vi "Display.vi"(8 "error in":errorcluster, 11 "Custom - Two Button in":refnum<class "Custom - Two Button.lvclass">) -> (0 "error out":errorcluster, 3 "Custom - Two Button out":refnum<class "Custom - Two Button.lvclass">)   [LabVIEW 2021, in "Pop-Up.lvlib" / "Custom - Two Button.lvclass"]
doc: "This VI will display a custom image to the user along with their message and buttons for pos/neg choice\n\n<b>Code Developed By:</b>\nDaniel Coons\nTechnology Service Corporation\n1983 S Liberty Drive\nBloomington, IN 47403\nPhone: 812 558-7100\ndaniel.coons@tsc.com\nwww.tsc.com/atcs"
uses:
  Custom - Two Button.lvclass
  C:/Development/Open Source/tsc-pop-up/Popup/Popup.lvclass
  <vilib>/Utility/miscctls.llb/LVPositionTypeDef.ctl
  Custom - Two Button.lvclass/Custom - Two Button.ctl
  Popup/Popup.lvclass/Popup.ctl
  Popup/Data Member Access/Read Theme.vi
  Theme/Theme.lvclass
  Popup/Popup.lvclass
  user32.dll
panel:
  out "header":bool
  in  "n-choice":bool
  in  "y-choice":bool
  out "2D Picture":picture
  out "Message":string
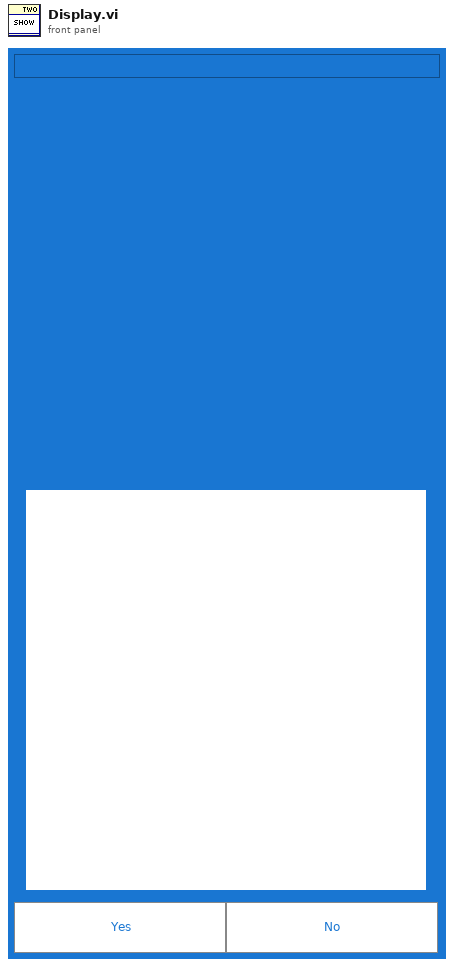
[diagram p1: front panel]
types:
  T1 = typedef "LVPositionTypeDef.ctl" = cluster{"Left":i32, "Top":i32}
  T2 = typedef "LVPoint32TypeDef.ctl" = cluster{"Horizontal":i32, "Vertical":i32}
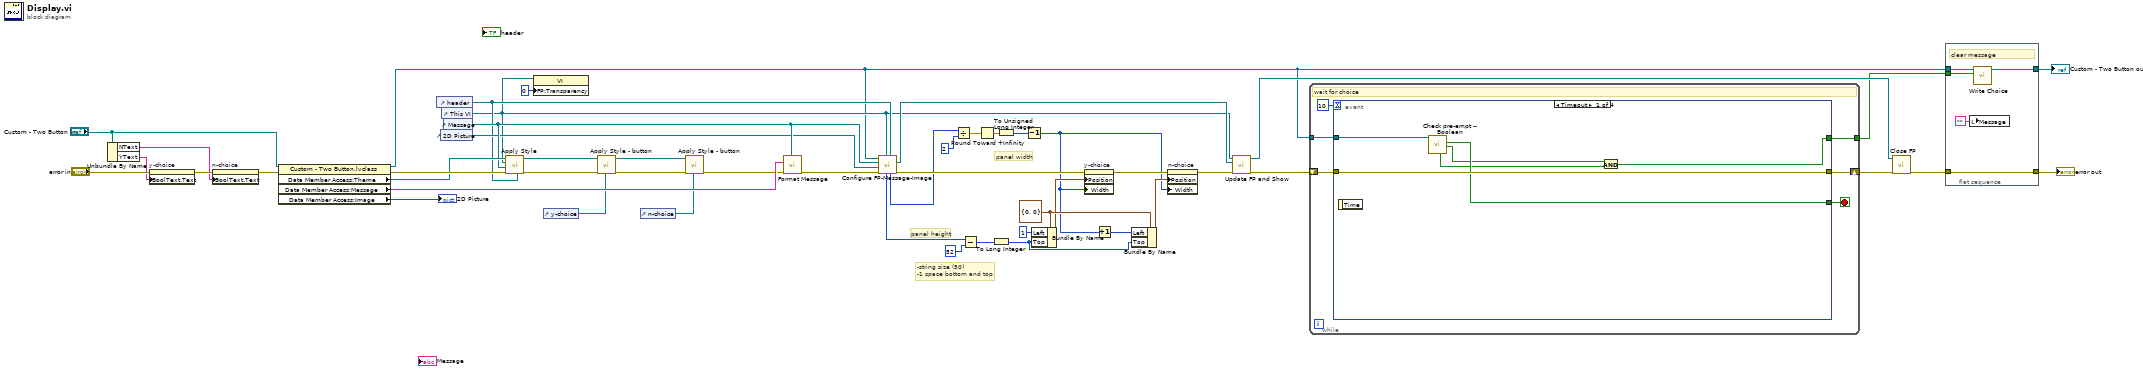
[diagram p0: block diagram]
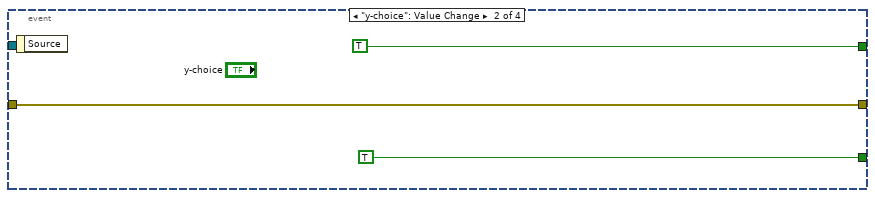
[diagram p2: hidden frame]
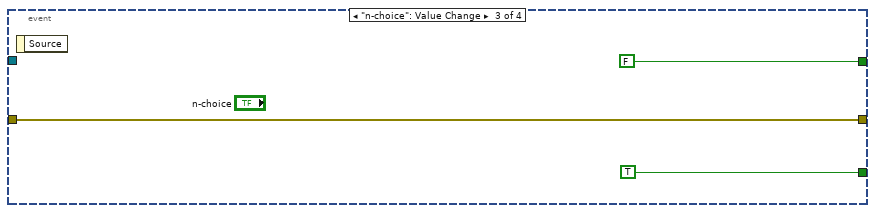
[diagram p3: hidden frame]
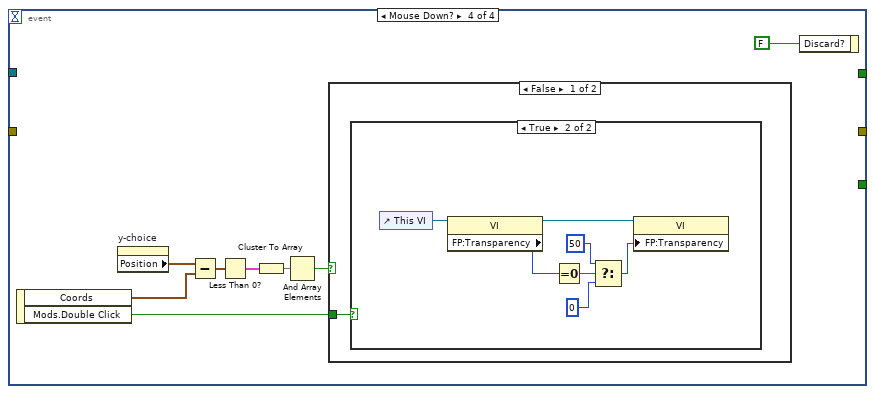
[diagram p4: hidden frame]
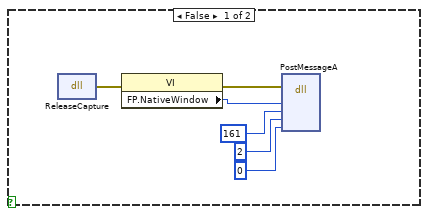
[diagram p5: hidden frame]
diagram:
  w37 = T1 {"Left"=0, "Top"=0} ("Position")
  # "-string size (50)\n-1 space bottom and top"
  # "panel width"
  # "panel height"
  n1 = Unbundle By Name("Custom - Two Button in") -> ("NText"=w39:string, "YText"=w42:string)
  n2 = property on="y-choice" class="Bool"(error in="error in", "BoolText.Text"=w42) -> (error out=w41:errorcluster)  [unwired: 1 in, 1 out]
  n3 = property on="n-choice" class="Bool"(error in=w41, "BoolText.Text"=w39) -> (error out=w40:errorcluster)  [unwired: 1 in, 1 out]
  n4 = property class="Custom - Two Button.lvclass"(reference="Custom - Two Button in", error in=w40) -> (reference out=w1:refnum<class "Custom - Two Button.lvclass">, error out=w24:errorcluster, "Data Member Access:Theme"=w22:refnum<class "Theme.lvclass">, "Data Member Access:Message"=w21:string, "Data Member Access:Image"=→"2D Picture":picture)
  n5 = control-ref of="header"() -> (w10:refnum<vi>)
  n6 = control-ref of="2D Picture"() -> (w11:refnum<vi>)
  n7 = control-ref of="This VI"() -> (w3:refnum<vi>)
  n8 = control-ref of="Message"() -> (w12:refnum<vi>)
  n9 = call "Apply Style.vi"("header ref"=w10, "error in"=w24, "message ref"=w12, "pop up ref"=w3, "Theme in"=w22) -> ("error out"=w23:errorcluster, "Theme out"=w16:refnum<class "Theme.lvclass">)  [unwired: 5 in]
  n10 = property class="VI"(reference=w3, "FP:Transparency"=u8 0 ("Front Panel Window:Transparency")) -> ()  [unwired: 1 in, 2 out]
  n11 = control-ref of="y-choice"() -> (w17:refnum<vi>)
  n12 = call "Apply Style - button.vi"("button ref"=w17, "error in"=w23, "Theme in"=w16) -> ("error out"=w19:errorcluster, "Theme out"=w14:refnum<class "Theme.lvclass">)  [unwired: 7 in]
  n13 = control-ref of="n-choice"() -> (w15:refnum<vi>)
  n14 = call "Apply Style - button.vi"("button ref"=w15, "error in"=w19, "Theme in"=w14) -> ("error out"=w20:errorcluster)  [unwired: 7 in, 1 out]
  n15 = call "Format Message.vi"("formatted string"=w12, "error in"=w20, "String Input"=w21) -> ("error out"=w13:errorcluster)  [unwired: 7 in, 1 out]
  n16 = call "Configure FP-Message-Image.vi"("header ref"=w10, "Pop Up ref"=w3, "error in (no error)"=w13, "Image ref"=w11, "Message ref"=w12, "Popup in"=w1) -> ("error out"=w8:errorcluster, "Panel Ref"=w7:refnum<vi>, "Panel Width"=w6:i32, "Panel Height"=w9:i32)  [unwired: 1 in, 1 out]
  n17 = Divide(x=w6, y=2) -> (x/y=w28:dbl)
  n18 = Subtract(x=w9, y=52 ("value")) -> (x-y=w32:i32)
  n19 = Round Toward +Infinity(x=w28) -> (ceil(x): smallest int >= x=w25:dbl)
  n20 = To Long Integer(number=w32) -> (32bit integer=w35:i32)
  n21 = To Unsigned Long Integer(number=w25) -> (unsigned 32bit integer=w26:u32)
  n22 = Decrement(x=w26) -> (x-1=w4:u32)
  n23 = Bundle By Name(cluster=w37, "Left"=1, "Top"=w35) -> (w33:T1)
  n24 = property on="y-choice" class="Bool"(error in=w8, "Position"=w33, "Width"=w4) -> (error out=w34:errorcluster)  [unwired: 1 in, 1 out]
  n25 = Increment(x=w4) -> (x+1=w5:u32)
  n26 = Bundle By Name(cluster=w37, "Left"=w5, "Top"=w35) -> (w36:T1)
  n27 = property on="n-choice" class="Bool"(error in=w34, "Position"=w36, "Width"=w4) -> (error out=w30:errorcluster)  [unwired: 1 in, 1 out]
  n28 = call "Update FP and Show.vi"("error in (no error)"=w30, "Panel Ref"=w7, "VI in"=w3) -> ("error out"=w45:errorcluster, "VI out"=w46:refnum<vi>)  [unwired: 7 in]
  n29 = while {
    tunnel: [w54] -> w38
    shift-right: [w56] -> w48
    shift-left: w45 -> [w55]
    tunnel: w1 -> [w51]
    stop <- w53 stop-if-true
    # "wait for choice"
    n30 = event shown="[0] Timeout" {
      selector: _ -> [_ _ _ _]
      dyn-events: _ -> [_ _ _ _]
      timeout: 10 -> [_ _ _ _]
      tunnel: w55 -> [w62 w65 w68 _]
      tunnel: [w62 w65 w68 _] -> w56
      tunnel: [w57 TRUE FALSE _] -> w54
      tunnel: [w60 TRUE TRUE _] -> w53
      tunnel: w51 -> [w61 _ _ _]
      event Timeout {
        n31 = event-data() -> ()  [unwired: 1 in, 1 out]
        n32 = call "Check pre-empt -- Boolean.vi"("_Popup in"=w61) -> ("Value?"=w59:bool, "Pre-empted?"=w60:bool, "Type Match?"=w58:bool)  [unwired: 7 in, 1 out]
        n33 = And(x=w59, y=w58) -> (x .and. y?=w57:bool)
      }
      event "y-choice": Value Change {
        n34 = event-data() -> ()  [unwired: 1 in, 1 out]
      }
      event "n-choice": Value Change {
        n35 = event-data() -> ()  [unwired: 1 in, 1 out]
      }
      event Mouse Down? {
        n36 = event-data() -> ("Coords"=w69:T2, "Mods.Double Click"=w70:bool)  [unwired: 1 in]
        n37 = property on="y-choice" class="Bool"() -> ("Position"=w75:T1)  [unwired: 2 in, 2 out]
        n38 = Subtract(x=w75, y=w69) -> (x-y=w74:T1)
        n39 = Less Than 0?(x=w74) -> (x < 0?=w73:cluster{"Left":bool, "Top":bool})
        n40 = Cluster To Array(cluster=w73) -> (array=w72:bool[])
        n41 = And Array Elements(Boolean array=w72) -> (logical AND=w71:bool)
        n42 = case shown="False" w71 {
          tunnel: w70 -> [w77 _]
          frame False {
            n43 = case shown="True" w77 {
              frame False {
                n44 = dll-call lib="user32.dll" fn="ReleaseCapture"() -> (error out=w81:errorcluster)  [unwired: 4 in, 1 out]
                n45 = property class="VI"(error in=w81) -> (error out=w82:errorcluster, "FP.NativeWindow"=w83:u64)  [unwired: 1 in, 1 out]
                n46 = dll-call lib="user32.dll" fn="PostMessageA"(error in=w82, "hWnd"=w83, "Msg"=161, "wParam"=2, "lParam"=0) -> ()  [unwired: 7 in, 2 out]
              }
              frame True {
                n47 = control-ref of="This VI"() -> (w90:refnum<vi>)
                n48 = property class="VI"(reference=w90) -> (reference out=w88:refnum<vi>, "FP:Transparency"=w89:u8)  [unwired: 1 in, 1 out]
                n49 = Equal To 0?(x=w89) -> (x = 0?=w87:bool)
                n50 = Select(t=u8 50, s=w87, f=u8 0) -> (s? t:f=w86:u8)
                n51 = property class="VI"(reference=w88, "FP:Transparency"=w86) -> ()  [unwired: 1 in, 2 out]
              }
            }
          }
          frame True {
          }
        }
        n52 = event-data("Discard?"=FALSE) -> ()  [unwired: 1 in, 1 out]
      }
    }
  }
  n53 = call "Close FP.vi"("error in (no error)"=w48, "VI in"=w46) -> ("error out"=w47:errorcluster)  [unwired: 9 in]
  n54 = flat-sequence {
    tunnel: w47 -> [w95]
    tunnel: [w95] -> w49
    tunnel: w1 -> [w94]
    tunnel: [w92] -> w50
    tunnel: w38 -> [w91]
    frame #0 {
      # "clear message"
      n55 = local write "Message"("" ("Message")) -> ()
      n56 = call-dynamic "Write Choice.vi"("Choice"=w91, "_Popup in"=w94) -> ("_Popup out"=w92:refnum<class "Custom - Two Button.lvclass">)  [unwired: 8 in, 1 out]
    }
  }
  "error out" <- w49
  "Custom - Two Button out" <- w50
